vi "Actor Core.vi"(8 "error in":errorcluster, 11 "Client Controller in":refnum<class "Client Controller.lvclass">) -> (0 "error out":errorcluster, 3 "Actor out":refnum<class "Actor.lvclass">)   [LabVIEW 2026, in "Client Controller.lvlib" / "Client Controller.lvclass"]
doc: "(<B>Filename</B>: Actor Framework.lvlib:Actor.lvclass:Actor Core.vi)\n\nReceives messages to the actor, reacts to them, and initiates any error handling that may shut the actor down.\n\nDescendant classes may override this VI to append parallel tasks for the actor to complete while it handles messages. Overrides use the Call Parent Method node."
uses:
  Client Controller.lvclass
  Client Controller.lvclass/Client Controller.ctl
  <vilib>/ActorFramework/Actor/Actor.lvclass/Actor.ctl
  <vilib>/ActorFramework/Message Enqueuer/Message Enqueuer.lvclass/Message Enqueuer.ctl
  C:/Users/E2013170/Documents/GitHub/Measurement-Utility-Reference/components/MAL-Framework/user.lib/Common Components/Controller/Controller.lvclass
  C:/Program Files/National Instruments/LabVIEW 2026/vi.lib/ActorFramework/Actor/Actor.lvclass
  C:/Users/E2013170/Documents/GitHub/Measurement-Utility-Reference/components/HAL-MAL-Application/Source/Framework/Client/Client Controller/Client Controller.lvclass
  Messages/Negotiate Server Connection Msg/Negotiate Server Connection Msg.lvclass
  MAL-Framework/user.lib/Common Components/Controller/Messages/Find Devices of Specified Type Msg/Find Devices of Specified Type Msg.lvclass
  MAL-Framework/user.lib/Common Components/Controller/Messages/Respond with Devices for Measurement Msg/Respond with Devices for Measurement Msg.lvclass
  MAL-Framework/user.lib/Common Components/Controller/Messages/Launch UI Message/Launch User Interface Msg.lvclass
  MAL-Framework/user.lib/Common Components/Controller/Messages/Populate Mesaurements in UI/Display Measurements Message.lvclass
  MAL-Framework/user.lib/Common Components/Controller/Messages/Find Compatible Hardware for Measurement Msg/Find Compatible Hardware for Measurement Msg.lvclass
  MAL-Framework/user.lib/Common Components/Controller/Messages/Load Measurements/Find Measurements On Disk Message.lvclass
  MAL-Framework/user.lib/Common Components/Controller/Messages/Launch Measurements Message/Launch Measurements Message.lvclass
  MAL-Framework/user.lib/Common Components/Controller/Messages/Launch Results UI Msg/Launch Results UI Msg.lvclass
  MAL-Framework/user.lib/Common Components/Controller/Messages/Log Status/Log Status.lvclass
  MAL-Framework/user.lib/Common Components/Controller/Messages/Measurement Done Message/Measurement Done.lvclass
  MAL-Framework/user.lib/Common Components/Controller/Messages/Scan Hardware Message/Scan Hardware Message.lvclass
  MAL-Framework/user.lib/Common Components/Controller/Messages/Send Results Object/Send Results Object.lvclass
  MAL-Framework/user.lib/Common Components/Controller/Messages/Add Available Measurement Msg/Add Available Measurement Msg.lvclass
  MAL-Framework/user.lib/Common Components/Hardware/DMM/DMM.lvclass
  MAL-Framework/user.lib/Common Components/Hardware/FGEN/Function Generator.lvclass
  MAL-Framework/user.lib/Common Components/Hardware/PSU/PSU.lvclass
  MAL-Framework/user.lib/Common Components/Hardware/Scope/Scope.lvclass
  Messages/Stop LNA Msg/Stop LNA Msg.lvclass
  <vilib>/ActorFramework/Actor/Actor.lvclass
  MAL-Framework/user.lib/Common Components/Controller/Controller.lvclass
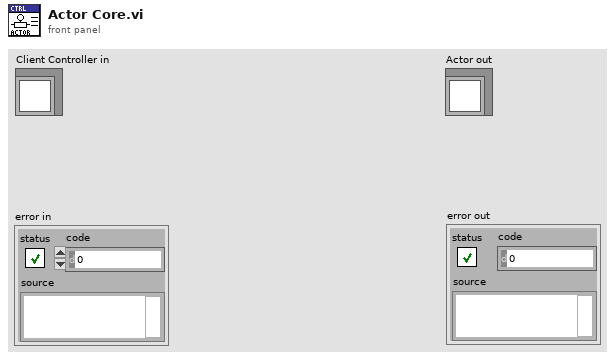
[diagram p1: front panel]
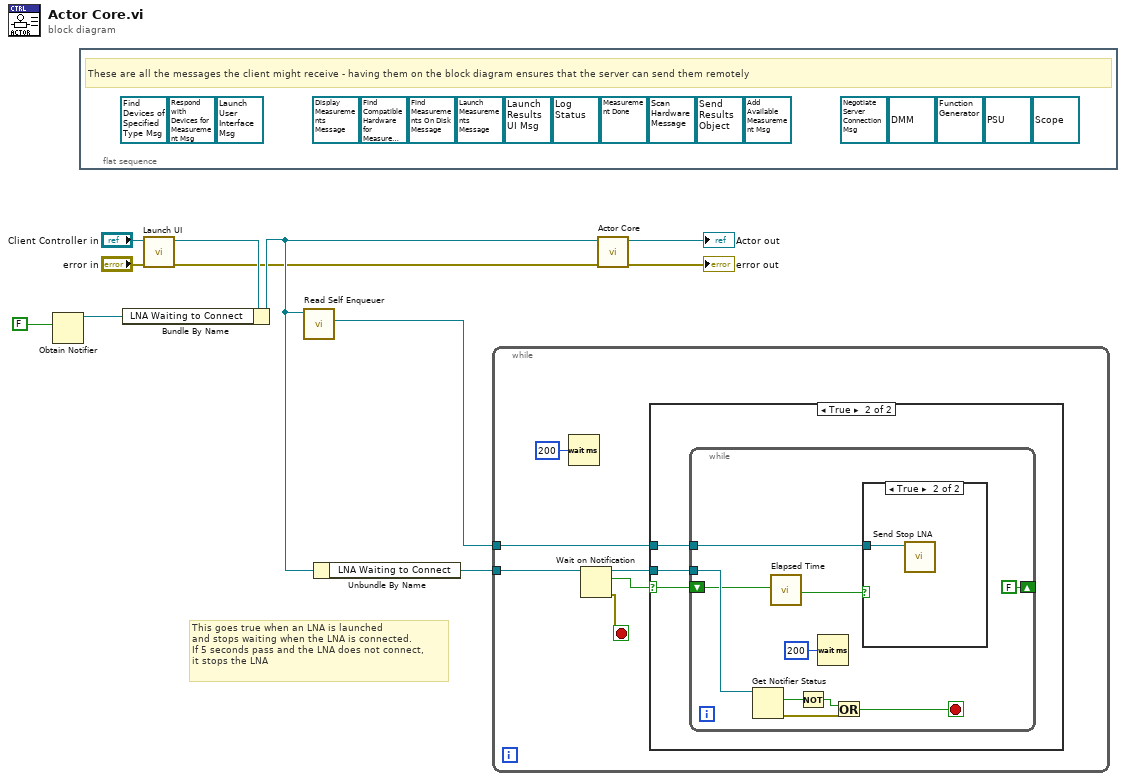
[diagram p0: block diagram]
diagram:
  # "This goes true when an LNA is launched\nand stops waiting when the LNA is connected.\nIf 5 seconds pass and the LNA does not connect,\nit stops the LNA"
  n1 = Obtain Notifier(notification data type=FALSE ("x .or. y?")) -> (notifier out=w5:refnum<notifier>)  [unwired: 3 in, 2 out]
  n2 = flat-sequence {
    frame #0 {
      (unwired) refnum<class "Scope.lvclass"> refnum ("Hardware.lvlib:Scope.lvclass")
      (unwired) refnum<class "PSU.lvclass"> refnum ("Hardware.lvlib:PSU.lvclass")
      (unwired) refnum<class "Function Generator.lvclass"> refnum ("Hardware.lvlib:Function Generator.lvclass")
      (unwired) refnum<class "DMM.lvclass"> refnum ("Hardware.lvlib:DMM.lvclass")
      (unwired) refnum<class "Add Available Measurement Msg.lvclass"> refnum ("Controller Actor.lvlib:Add Available Measurement Msg.lvclass")
      (unwired) refnum<class "Send Results Object.lvclass"> refnum ("Controller Actor.lvlib:Send Results Object.lvclass")
      (unwired) refnum<class "Scan Hardware Message.lvclass"> refnum ("Controller Actor.lvlib:Scan Hardware Message.lvclass")
      (unwired) refnum<class "Measurement Done.lvclass"> refnum ("Controller Actor.lvlib:Measurement Done.lvclass")
      (unwired) refnum<class "Log Status.lvclass"> refnum ("Controller Actor.lvlib:Log Status.lvclass")
      (unwired) refnum<class "Launch Results UI Msg.lvclass"> refnum ("Controller Actor.lvlib:Launch Results UI Msg.lvclass")
      (unwired) refnum<class "Launch Measurements Message.lvclass"> refnum ("Controller Actor.lvlib:Launch Measurements Message.lvclass")
      (unwired) refnum<class "Find Measurements On Disk Message.lvclass"> refnum ("Controller Actor.lvlib:Find Measurements On Disk Message.lvclass")
      (unwired) refnum<class "Find Compatible Hardware for Measurement Msg.lvclass"> refnum ("Controller Actor.lvlib:Find Compatible Hardware for Measurement Msg.lvclass")
      (unwired) refnum<class "Display Measurements Message.lvclass"> refnum ("Controller Actor.lvlib:Display Measurements Message.lvclass")
      (unwired) refnum<class "Launch User Interface Msg.lvclass"> refnum ("Controller Actor.lvlib:Launch User Interface Msg.lvclass")
      (unwired) refnum<class "Respond with Devices for Measurement Msg.lvclass"> refnum ("Controller Actor.lvlib:Respond with Devices for Measurement Msg.lvclass")
      (unwired) refnum<class "Find Devices of Specified Type Msg.lvclass"> refnum ("Controller Actor.lvlib:Find Devices of Specified Type Msg.lvclass")
      (unwired) refnum<class "Negotiate Server Connection Msg.lvclass"> refnum ("Client Controller.lvlib:Negotiate Server Connection Msg.lvclass")
      # "These are all the messages the client might receive - having them on the block diagram ensures that the server can send them remotely"
    }
  }
  n3 = call-dynamic "Launch UI.vi"("error in (no error)"="error in", "Controller In"="Client Controller in") -> ("error out"=w3:errorcluster, "Controller Out"=w4:refnum<class "Client Controller.lvclass">)  [unwired: 8 in]
  n4 = Bundle By Name(cluster=w4, "LNA Waiting to Connect"=w5) -> (w7:refnum<class "Client Controller.lvclass">)
  n5 = call <vilib>:"Read Self Enqueuer.vi"("Actor"=w7) -> ("Self Enqueuer"=w9:refnum<class "Message Enqueuer.lvclass">)  [unwired: 10 in]
  n6 = Unbundle By Name(w7) -> ("LNA Waiting to Connect"=w8:refnum<notifier>)
  n7 = while {
    tunnel: w8 -> [w15]
    tunnel: w9 -> [w16]
    stop <- w12 stop-if-true
    n8 = Wait (ms)(milliseconds to wait=u32 200) -> ()  [unwired: 1 out]
    n9 = Wait on Notification(notifier=w15) -> (notifier out=w14:refnum<notifier>, notification=w13:bool, error out=w12:errorcluster)  [unwired: 3 in, 1 out]
    n10 = case shown="True" w13 {
      selector: w13 -> [_ w18]
      tunnel: w14 -> [_ w20]
      tunnel: w16 -> [_ w19]
      frame False {
      }
      frame True {
        n11 = while {
          tunnel: w20 -> [w29]
          tunnel: w19 -> [w27]
          shift-right: [FALSE] -> _
          shift-left: w18 -> [w22]
          stop <- w25 stop-if-true
          n12 = Get Notifier Status(notifier=w29) -> (current notification=w24:bool, error out=w26:errorcluster)  [unwired: 1 in, 3 out]
          n13 = call "Elapsed Time"("Reset"=w22) -> ("Time has Elapsed"=w30:bool)  [unwired: 11 in, 7 out]
          n14 = Not(x=w24) -> (.not. x?=w23:bool)
          n15 = Wait (ms)(milliseconds to wait=u32 200) -> ()  [unwired: 1 out]
          n16 = Or(x=w23, y=w26) -> (x .or. y?=w25:bool)
          n17 = case shown="True" w30 {
            tunnel: w27 -> [_ w31]
            frame False {
            }
            frame True {
              n18 = call "Send Stop LNA.vi"("Message Enqueuer"=w31) -> ()  [unwired: 9 in, 2 out]
            }
          }
        }
      }
    }
  }
  n19 = call-parent "Actor Core.vi"("error in"=w3, "Controller in"=w7) -> ("error out"=→"error out":errorcluster, "Actor out"=→"Actor out":refnum<class "Actor.lvclass">)  [unwired: 8 in]
